vi "_Persist New Entity.vi"(8 "error in (no error)":errorcluster, 9 "Entity":refnum<class "Entity.lvclass">, 10 "Types":refnum<class "Type.lvclass">[](array[class]), 11 "Database in":refnum<class "Database Platform.lvclass">) -> (0 "error out":errorcluster, 2 "New ID":T1, 3 "Database out":refnum<class "Database Platform.lvclass">)   [LabVIEW 2020, in "Conditu2.lvlib" / "Database Platform.lvclass"]
uses:
  Database Platform.lvclass
  Entity/Entity.lvclass
  Entity ID.ctl
  Columns/Type/Type.lvclass
  Columns/Relation/Validate Persistance.vi
  Columns/Relation/Relation.lvclass
  Conditu2.lvlib
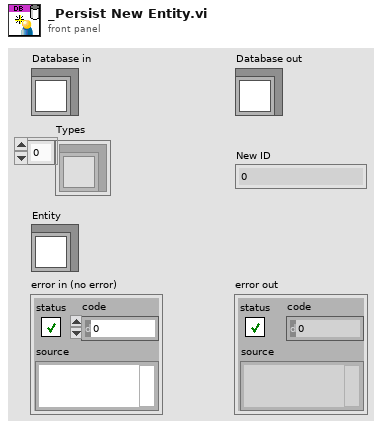
[diagram p1: front panel]
types:
  T1 = typedef "Conditu2.lvlib/Entity ID.ctl" = i64
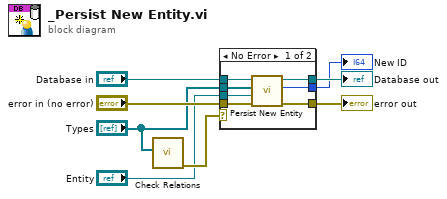
[diagram p0: block diagram]
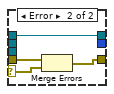
[diagram p2: hidden frame]
diagram:
  n1 = call "Check Relations.vi"("Types"="Types") -> ("error out"=w8:errorcluster)  [unwired: 10 in]
  n2 = case shown="No Error" w8 {
    selector: w8 -> [_ w18]
    tunnel: "Database in" -> [w15 w16]
    tunnel: "error in (no error)" -> [w14 w19]
    tunnel: [w13 w17] -> w5
    tunnel: "Entity" -> [w12 _]
    tunnel: [w11 w16] -> w3
    tunnel: [w10 _] -> w2
    tunnel: "Types" -> [w9 _]
    frame No Error {
      n3 = call-dynamic "Persist New Entity.vi"("error in (no error)"=w14, "Entity"=w12, "Types"=w9, "Database in"=w15) -> ("error out"=w13:errorcluster, "New ID"=w10:T1, "Database out"=w11:refnum<class "Database Platform.lvclass">)  [unwired: 5 in]
    }
    frame Error {
      n4 = Merge Errors(w19, w18) -> (w17:errorcluster)
    }
  }
  "error out" <- w5
  "Database out" <- w3
  "New ID" <- w2
